vi "Set DAC.vi"(0 "DAC":u32, 2 "Channel Number":i16) -> ()   [LabVIEW 2018]
uses:
  <vilib>/rvi/eio/common/nirviEmuTemplateMethod_errors.vi
  <vilib>/eio/EIONode/EIONode.xnode
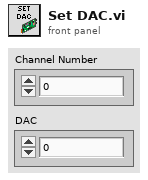
[diagram p1: front panel]
types:
  T1 = cluster{"Boolean array[0]":bool, "Boolean array[1]":bool, "Boolean array[2]":bool, "Boolean array[3]":bool, "Boolean array[4]":bool, "Boolean array[5]":bool, "Boolean array[6]":bool, "Boolean array[7]":bool, "Boolean array[8]":bool, "Boolean array[9]":bool, "Boolean array[10]":bool, "Boolean array[11]":bool, "Boolean array[12]":bool, "Boolean array[13]":bool, "Boolean array[14]":bool, "Boolean array[15]":bool, "Boolean array[16]":bool, "Boolean array[17]":bool, "Boolean array[18]":bool, "Boolean array[19]":bool, "Boolean array[20]":bool, "Boolean array[21]":bool, "Boolean array[22]":bool, "Boolean array[23]":bool, "Boolean array[24]":bool, "Boolean array[25]":bool, "Boolean array[26]":bool, "Boolean array[27]":bool, "Boolean array[28]":bool, "Boolean array[29]":bool, "Boolean array[30]":bool, "Boolean array[31]":bool}
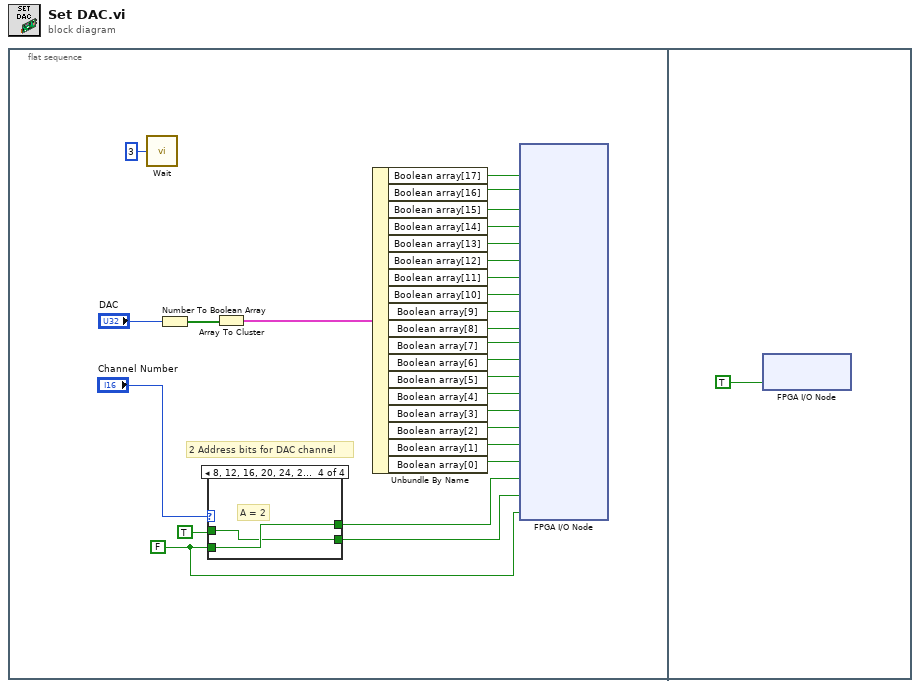
[diagram p0: block diagram]
diagram:
  n1 = flat-sequence {
    frame #0 {
      w2 = FALSE
      # "2 Address bits for DAC channel"
      n2 = call "Wait"("Count(Ticks)"=u8 3) -> ()  [unwired: 1 out]
      n3 = Number To Boolean Array(number="DAC") -> (Boolean array=w26:bool[])
      n4 = case shown="8, 12, 16, 20, 24, 28, 42" "Channel Number" {
        tunnel: TRUE -> [w28 _ w31 w32]
        tunnel: w2 -> [_ w29 w30 w33]
        tunnel: [w28 w29 w31 w33] -> w6
        tunnel: [w28 w29 w30 w32] -> w5
        frame 1, Default {
          # "A = 3"
        }
        frame 6, 10, 14, 18, 22, 26, 30 {
          # "A = 0"
        }
        frame 7, 11, 15, 19, 23, 27, 31 {
          # "A = 1"
        }
        frame 8, 12, 16, 20, 24, 28, 42 {
          # "A = 2"
        }
      }
      n5 = Array To Cluster(array=w26) -> (cluster=w25:T1)
      n6 = Unbundle By Name(w25) -> ("Boolean array[17]"=w24:bool, "Boolean array[16]"=w23:bool, "Boolean array[15]"=w22:bool, "Boolean array[14]"=w21:bool, "Boolean array[13]"=w20:bool, "Boolean array[12]"=w19:bool, "Boolean array[11]"=w18:bool, "Boolean array[10]"=w17:bool, "Boolean array[9]"=w16:bool, "Boolean array[8]"=w15:bool, "Boolean array[7]"=w14:bool, "Boolean array[6]"=w13:bool, "Boolean array[5]"=w12:bool, "Boolean array[4]"=w11:bool, "Boolean array[3]"=w10:bool, "Boolean array[2]"=w9:bool, "Boolean array[1]"=w8:bool, "Boolean array[0]"=w7:bool)
      n7 = xnode "FPGA I/O Node"("D17"=w24, "D16"=w23, "D15"=w22, "D14"=w21, "D13"=w20, "D12"=w19, "D11"=w18, "D10"=w17, "D9"=w16, "D8"=w15, "D7"=w14, "D6"=w13, "D5"=w12, "D4"=w11, "D3"=w10, "D2"=w9, "D1"=w8, "D0"=w7, "DAC A0"=w6, "DAC A1"=w5, "DAC WR"=w2) -> ()  [unwired: 21 in, 21 out]
    }
    frame #1 {
      n8 = xnode "FPGA I/O Node"("DAC WR"=TRUE) -> ()  [unwired: 1 in, 1 out]
    }
  }
